vi "ASK_BitAllocation.vi"(0 "PathIn":path, 5 "code_model":i32, 7 "n":i32, 9 "Origin_Bit":dbl[](array[numeric]) format="%#_13g", 11 "error in (no error)":errorcluster caption="错误输入（无错误）") -> (4 "PathOut":path, 6 "paddingBits":i32, 8 "FreData":dbl[][](array[numeric]), 10 "frame_num":i32, 14 "bitLen":dbl format="%#_13g", 15 "error out":errorcluster caption="错误输出")   [LabVIEW 2015]
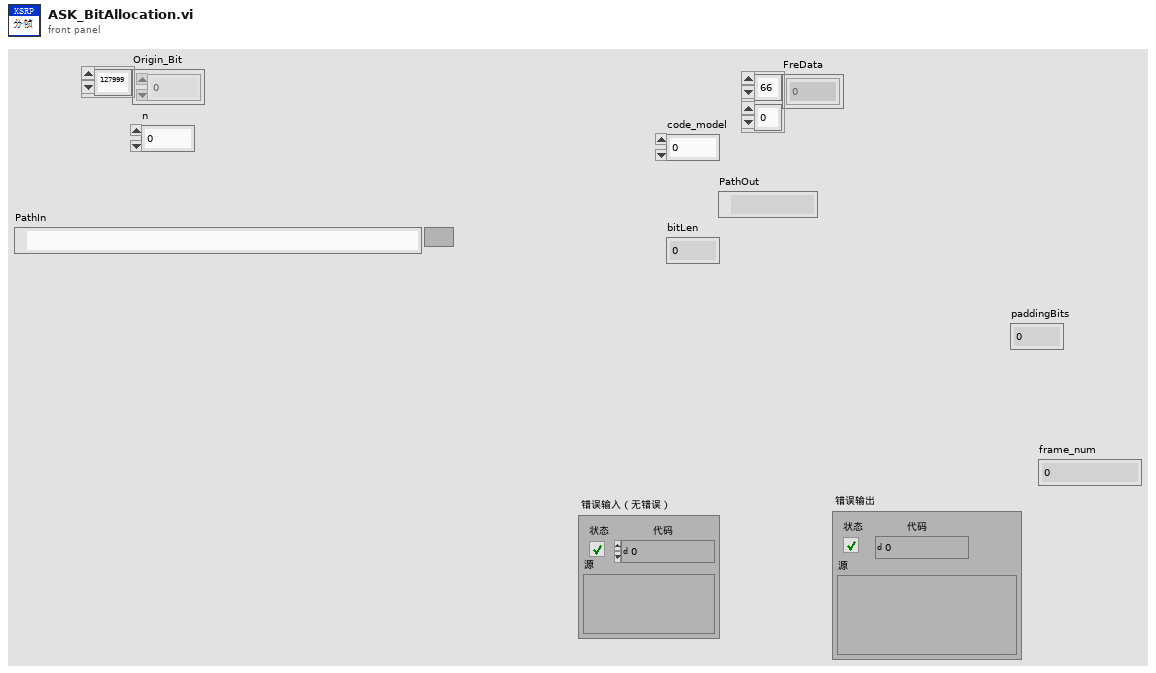
[diagram p1: front panel]
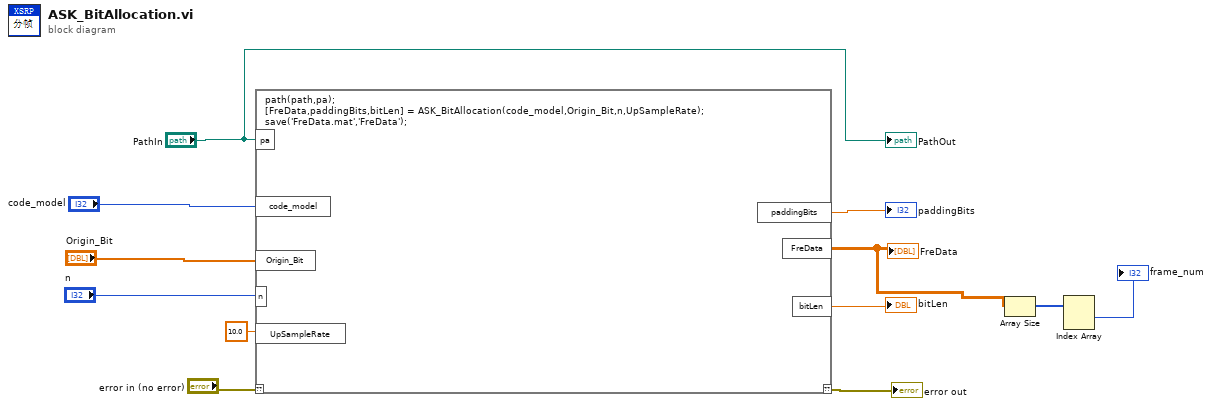
[diagram p0: block diagram]
diagram:
  n1 = script code="path(path,pa);\n[FreData,paddingBits,bitLen] = ASK_BitAllocation(code_model,Origin_Bit,n,UpSampleRate);\nsave('FreData.mat','FreData');"("??"="error in (no error)", "pa"="PathIn", "code_model"="code_model", "Origin_Bit"="Origin_Bit", "n"="n", "UpSampleRate"=10.0 ("Real")) -> ("??"=→"error out":errorcluster, "paddingBits"=→"paddingBits":dbl, "FreData"=w4:dbl[][], "bitLen"=→"bitLen":dbl)
  "FreData" <- w4
  n2 = Array Size(array=w4) -> (size(s)=w3:i32[])
  n3 = Index Array(array=w3) -> (element #1=→"frame_num":i32)  [unwired: 2 in, 1 out]
  "PathOut" <- "PathIn"
